vi "update.vi"(8 "error in (no error)":errorcluster, 11 "TrajectoryRK110428Fiber in":refnum<class "TrajectoryRK110428Fiber_Spiral.lvclass">) -> (0 "error out":errorcluster, 3 "TrajectoryRK110428Fiber out":refnum<class "TrajectoryRK110428Fiber_Spiral.lvclass">)   [LabVIEW 2010, in "TrajectoryRK110428Fiber_Spiral.lvclass"]
uses:
  TrajectoryRK110428Fiber_Spiral.lvclass
  FPGAWrapper/GenericFPGAWrapper/GenericFPGAWrapper/GenericFPGAWrapper.lvclass
  FPGAWrapper/FPGAWrapperRK110512Fiber/FPGAWrapperRK110512Fiber_Spiral/FPGAWrapperRK110512Fiber_Spiral.lvclass
  TrajectoryRK110428Fiber_Spiral.lvclass/TrajectoryRK110428Fiber_Spiral.ctl
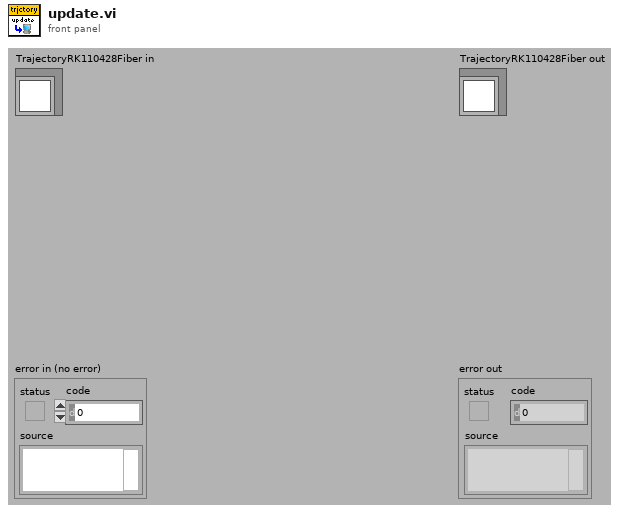
[diagram p1: front panel]
types:
  T1 = typedef "FPGAWrapperRK110512Fiber_Spiral.lvclass/fiber_spiral_parameters.ctl" = cluster{"Fiber Frequency":u16, "Imaging Periods":u16, "Settling Periods":u16, "Resting Periods":u16, "Amplitude X":dbl, "Amplitude Y":dbl, "Phase difference":dbl, "Initial Amplitude X":dbl, "Initial Amplitude Y":dbl}
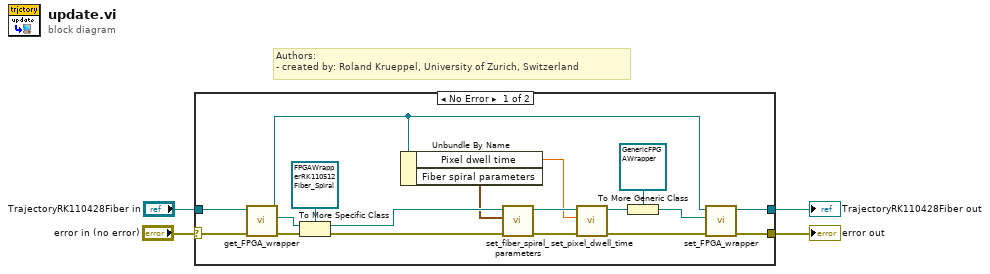
[diagram p0: block diagram]
diagram:
  # "Authors: \n- created by: Roland Krueppel, University of Zurich, Switzerland"
  n1 = case shown="No Error" "error in (no error)" {
    selector: "error in (no error)" -> [w22 w23]
    tunnel: "TrajectoryRK110428Fiber in" -> [w21 w24]
    tunnel: [w11 w24] -> w2
    tunnel: [w10 w23] -> w1
    frame No Error {
      n2 = call-dynamic "get_FPGA_wrapper.vi"("error in (no error)"=w22, "TrajectoryMG100122GenericFPGA in"=w21) -> ("error out"=w20:errorcluster, "GenericFPGAWrapper.lvclass"=w19:refnum<class "GenericFPGAWrapper.lvclass">, "TrajectoryMG100122GenericFPGA out"=w12:refnum<class "TrajectoryRK110428Fiber_Spiral.lvclass">)  [unwired: 7 in]
      n3 = To More Specific Class(target class=refnum<class "FPGAWrapperRK110512Fiber_Spiral.lvclass"> refnum ("FPGAWrapperRK110512Fiber_Spiral.lvclass"), reference=w19, error in=w20) -> (specific class reference=w16:refnum<class "FPGAWrapperRK110512Fiber_Spiral.lvclass">, error out=w17:errorcluster)
      n4 = Unbundle By Name(w12) -> ("Pixel dwell time"=w5:dbl, "Fiber spiral parameters"=w15:T1)
      n5 = call-dynamic "set_fiber_spiral_parameters.vi"("error in (no error)"=w17, "Fiber spiral parameters"=w15, "FPGAWrapperRK120511Fiber_Spiral in"=w16) -> ("error out"=w8:errorcluster, "FPGAWrapperRK120511Fiber_Spiral out"=w7:refnum<class "FPGAWrapperRK110512Fiber_Spiral.lvclass">)  [unwired: 7 in]
      n6 = call-dynamic "set_pixel_dwell_time.vi"("error in (no error)"=w8, "Pixel dwell time"=w5, "FPGAWrapperRK110512Fiber_Spiral in"=w7) -> ("error out"=w9:errorcluster, "FPGAWrapperRK110512Fiber_Spiral out"=w6:refnum<class "FPGAWrapperRK110512Fiber_Spiral.lvclass">)  [unwired: 7 in]
      n7 = To More Generic Class(target class=refnum<class "GenericFPGAWrapper.lvclass"> refnum ("GenericFPGAWrapper.lvclass"), reference=w6) -> (generic class reference=w13:refnum<class "GenericFPGAWrapper.lvclass">)
      n8 = call-dynamic "set_FPGA_wrapper.vi"("error in (no error)"=w9, "GenericFPGAWrapper.lvclass"=w13, "TrajectoryMG100122GenericFPGA in"=w12) -> ("error out"=w10:errorcluster, "TrajectoryMG100122GenericFPGA out"=w11:refnum<class "TrajectoryRK110428Fiber_Spiral.lvclass">)  [unwired: 7 in]
    }
    frame Error {
    }
  }
  "error out" <- w1
  "TrajectoryRK110428Fiber out" <- w2
